vi "NiSwitch RouteTriggerInput.vi"(6 "contextId":T1, 8 "error in":errorcluster, 9 "timeout (ms)":i32=-1, 10 "Request Data":T3, 11 "gRPC ID":T1) -> (0 "error out":errorcluster, 2 "Response Data":T2, 3 "gRPC ID out":T1)   [LabVIEW 2021, in "NI Switch_client.lvlib"]
uses:
  NI Switch_client.lvlib
  <vilib>/gRPC/LabVIEW gRPC Library/Shared/grpcId.ctl
  RPC Messages/niswitch_grpc_RouteTriggerInputRequest.ctl
  RPC Messages/niswitch_grpc_RouteTriggerInputRequest_trigger_input_connector_enum/niswitch_grpc_RouteTriggerInputRequest_trigger_input_connector_enum.lvclass
  RPC Messages/niswitch_grpc_RouteTriggerInputRequest_trigger_input_bus_line_enum/niswitch_grpc_RouteTriggerInputRequest_trigger_input_bus_line_enum.lvclass
  RPC Messages/nidevice_grpc_Session.ctl
  RPC Messages/niswitch_grpc_RouteTriggerInputResponse.ctl
  RPC Messages/niswitch_grpc_RouteTriggerInputResponse_Flat.ctl
  RPC Messages/niswitch_grpc_RouteTriggerInputRequest_trigger_input_connector_enum/niswitch_grpc_RouteTriggerInputRequest_trigger_input_connector_enum.lvclass/niswitch_grpc_RouteTriggerInputRequest_trigger_input_connector_enum.ctl
  RPC Messages/niswitch_grpc_RouteTriggerInputRequest_trigger_input_bus_line_enum/niswitch_grpc_RouteTriggerInputRequest_trigger_input_bus_line_enum.lvclass/niswitch_grpc_RouteTriggerInputRequest_trigger_input_bus_line_enum.ctl
  14035477-4c25-4107-8ed5-d0c4ef420ce5.vi
  RPC Messages/RichToFlatnidevice_grpc_Session.vi
  RPC Messages/niswitch_grpc_RouteTriggerInputRequest_trigger_input_connector_enum/GetActiveFieldIndex.vi
  RPC Messages/niswitch_grpc_RouteTriggerInputRequest_trigger_input_connector_enum/Gettrigger_input_connector.vi
  RPC Messages/niswitch_grpc_RouteTriggerInputRequest_trigger_input_connector_enum/Gettrigger_input_connector_raw.vi
  RPC Messages/niswitch_grpc_RouteTriggerInputRequest_trigger_input_bus_line_enum/GetActiveFieldIndex.vi
  RPC Messages/niswitch_grpc_RouteTriggerInputRequest_trigger_input_bus_line_enum/Gettrigger_input_bus_line.vi
  RPC Messages/niswitch_grpc_RouteTriggerInputRequest_trigger_input_bus_line_enum/Gettrigger_input_bus_line_raw.vi
  <vilib>/gRPC/LabVIEW gRPC Library/Shared/TranslateGrpcError.vi
  <vilib>/gRPC/LabVIEW gRPC Library/Shared/Wait On Occurrence Wrapper.vi
  <vilib>/gRPC/LabVIEW gRPC Library/Shared/Wait On Occurence.vi
  <vilib>/gRPC/LabVIEW gRPC Library/Server API/Server/Get Server DLL Path.vi
  <vilib>/Utility/error.llb/Error Cluster From Error Code.vi
  <vilib>/Utility/config.llb/Open Config Data.vi
  <vilib>/Utility/config.llb/Write Key.vi
  <vilib>/Utility/config.llb/Write Key (Boolean).vi
  <vilib>/Utility/config.llb/Not A Config Data Refnum.vi
  <vilib>/Utility/config.llb/Read Key.vi
  <vilib>/Utility/config.llb/Read Key (Boolean).vi
  <vilib>/Utility/config.llb/Close Config Data.vi
  <vilib>/gRPC/LabVIEW gRPC Library/grpc-lvsupport-release.lvlib
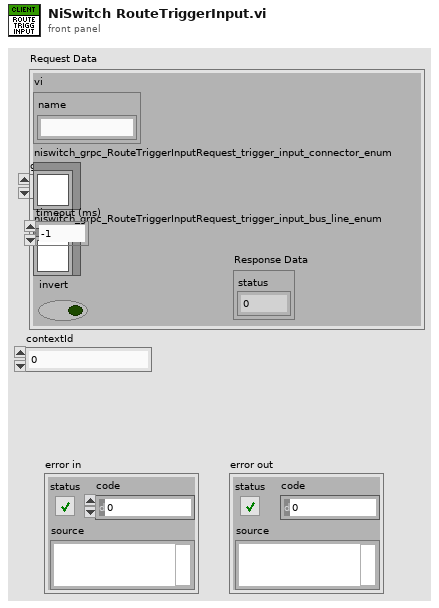
[diagram p1: front panel]
types:
  T1 = typedef "grpc-lvsupport-release.lvlib/grpcId.ctl" = u64
  T2 = typedef "NI Switch_client.lvlib/niswitch_grpc_RouteTriggerInputResponse.ctl" = cluster{"status":i32}
  T3 = typedef "NI Switch_client.lvlib/niswitch_grpc_RouteTriggerInputRequest.ctl" = cluster{"vi":T4, "niswitch_grpc_RouteTriggerInputRequest_trigger_input_connector_enum":refnum<class "niswitch_grpc_RouteTriggerInputRequest_trigger_input_connector_enum.lvclass">, "niswitch_grpc_RouteTriggerInputRequest_trigger_input_bus_line_enum":refnum<class "niswitch_grpc_RouteTriggerInputRequest_trigger_input_bus_line_enum.lvclass">, "invert":bool}
  T4 = typedef "NI Switch_client.lvlib/nidevice_grpc_Session.ctl" = cluster{"name":string}
  T5 = typedef "NI Switch_client.lvlib/niswitch_grpc_RouteTriggerInputResponse_Flat.ctl" = cluster{"status":i32}
  T6 = typedef "NI Switch_client.lvlib/niswitch_grpc_RouteTriggerInputRequest_Flat.ctl" = cluster{"vi":T7, "niswitch_grpc_RouteTriggerInputRequest_trigger_input_connector_enum_selected_index":i32, "trigger_input_connector":T8, "trigger_input_connector_raw":i32, "niswitch_grpc_RouteTriggerInputRequest_trigger_input_bus_line_enum_selected_index":i32, "trigger_input_bus_line":T8, "trigger_input_bus_line_raw":i32, "invert":bool}
  T7 = typedef "NI Switch_client.lvlib/nidevice_grpc_Session_Flat.ctl" = cluster{"name":string}
  T8 = typedef "NI Switch_client.lvlib/niswitch_grpc_TriggerInput.ctl" = enum32{"TRIGGER_INPUT_UNSPECIFIED", "TRIGGER_INPUT_NISWITCH_VAL_IMMEDIATE", "TRIGGER_INPUT_NISWITCH_VAL_EXTERNAL", "TRIGGER_INPUT_NISWITCH_VAL_SOFTWARE_TRIG", "TRIGGER_INPUT_NISWITCH_VAL_TTL0", "TRIGGER_INPUT_NISWITCH_VAL_TTL1", "TRIGGER_INPUT_NISWITCH_VAL_TTL2", "TRIGGER_INPUT_NISWITCH_VAL_TTL3", "TRIGGER_INPUT_NISWITCH_VAL_TTL4", "TRIGGER_INPUT_NISWITCH_VAL_TTL5", "TRIGGER_INPUT_NISWITCH_VAL_TTL6", "TRIGGER_INPUT_NISWITCH_VAL_TTL7", "TRIGGER_INPUT_NISWITCH_VAL_PXI_STAR", "TRIGGER_INPUT_NISWITCH_VAL_REARCONNECTOR", "TRIGGER_INPUT_NISWITCH_VAL_FRONTCONNECTOR", "TRIGGER_INPUT_NISWITCH_VAL_REARCONNECTOR_MODULE1", "TRIGGER_INPUT_NISWITCH_VAL_REARCONNECTOR_MODULE2", "TRIGGER_INPUT_NISWITCH_VAL_REARCONNECTOR_MODULE3", "TRIGGER_INPUT_NISWITCH_VAL_REARCONNECTOR_MODULE4", "TRIGGER_INPUT_NISWITCH_VAL_REARCONNECTOR_MODULE5", "TRIGGER_INPUT_NISWITCH_VAL_REARCONNECTOR_MODULE6", "TRIGGER_INPUT_NISWITCH_VAL_REARCONNECTOR_MODULE7", "TRIGGER_INPUT_NISWITCH_VAL_REARCONNECTOR_MODULE8", "TRIGGER_INPUT_NISWITCH_VAL_REARCONNECTOR_MODULE9", "TRIGGER_INPUT_NISWITCH_VAL_REARCONNECTOR_MODULE10", "TRIGGER_INPUT_NISWITCH_VAL_REARCONNECTOR_MODULE11", "TRIGGER_INPUT_NISWITCH_VAL_REARCONNECTOR_MODULE12", "TRIGGER_INPUT_NISWITCH_VAL_FRONTCONNECTOR_MODULE1", "TRIGGER_INPUT_NISWITCH_VAL_FRONTCONNECTOR_MODULE2", "TRIGGER_INPUT_NISWITCH_VAL_FRONTCONNECTOR_MODULE3", "TRIGGER_INPUT_NISWITCH_VAL_FRONTCONNECTOR_MODULE4", "TRIGGER_INPUT_NISWITCH_VAL_FRONTCONNECTOR_MODULE5", "TRIGGER_INPUT_NISWITCH_VAL_FRONTCONNECTOR_MODULE6", "TRIGGER_INPUT_NISWITCH_VAL_FRONTCONNECTOR_MODULE7", "TRIGGER_INPUT_NISWITCH_VAL_FRONTCONNECTOR_MODULE8", "TRIGGER_INPUT_NISWITCH_VAL_FRONTCONNECTOR_MODULE9", "TRIGGER_INPUT_NISWITCH_VAL_FRONTCONNECTOR_MODULE10", "TRIGGER_INPUT_NISWITCH_VAL_FRONTCONNECTOR_MODULE11", "TRIGGER_INPUT_NISWITCH_VAL_FRONTCONNECTOR_MODULE12"}
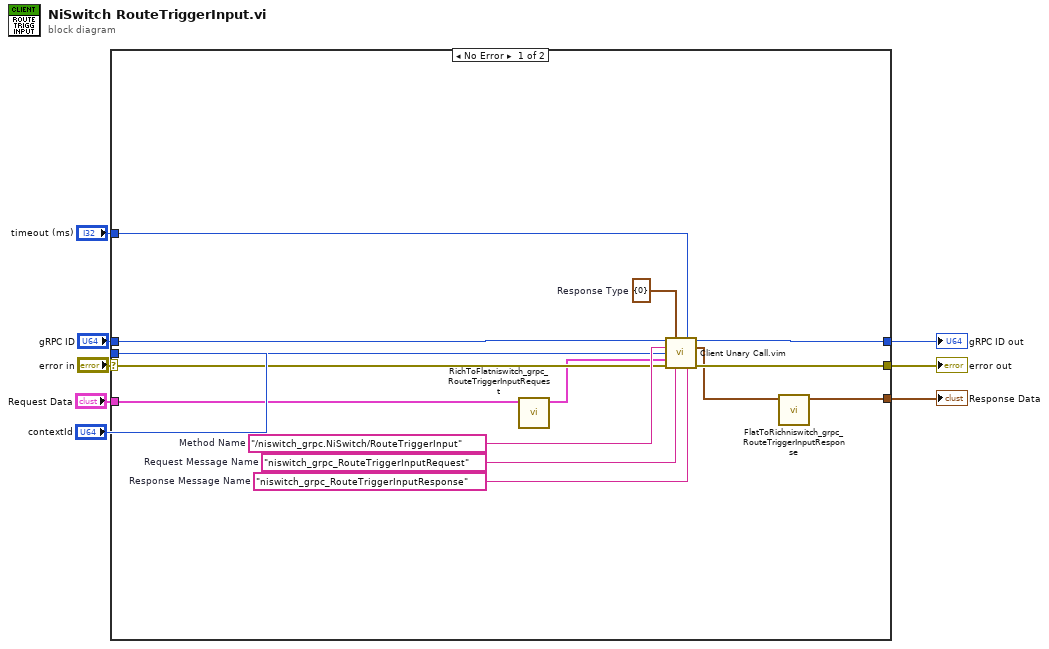
[diagram p0: block diagram]
diagram:
  n1 = case shown="No Error" "error in" {
    selector: "error in" -> [w18 w23]
    tunnel: [w17 w23] -> w7
    tunnel: "gRPC ID" -> [w16 w24]
    tunnel: [w15 w24] -> w5
    tunnel: "Request Data" -> [w12 _]
    tunnel: [w9 _] -> w3
    tunnel: "timeout (ms)" -> [w14 _]
    tunnel: "contextId" -> [w13 _]
    frame No Error {
      w19 = "niswitch_grpc_RouteTriggerInputResponse"  # Response Message Name
      w20 = "niswitch_grpc_RouteTriggerInputRequest"  # Request Message Name
      w21 = T5 {"status"=0}  # Response Type
      w22 = "/niswitch_grpc.NiSwitch/RouteTriggerInput"  # Method Name
      n2 = call "RichToFlatniswitch_grpc_RouteTriggerInputRequest.vi"("InputCluster"=w12) -> ("OutputCluster"=w11:T6)  [unwired: 10 in]
      n3 = call "Client Unary Call.vim"("ClientID in"=w16, "Response Type"=w21, "timeout (ms)"=w14, "Method Name"=w22, "contextId"=w13, "Request Data"=w11, "error in"=w18, "Request Message Name"=w20, "Response Message Name"=w19) -> ("ClientID out"=w15:u64, "Response Data"=w10:T5, "error out"=w17:errorcluster)  [unwired: 4 in]
      n4 = call "FlatToRichniswitch_grpc_RouteTriggerInputResponse.vi"("InputCluster"=w10) -> ("OutputCluster"=w9:T2)  [unwired: 10 in]
    }
    frame Error {
    }
  }
  "error out" <- w7
  "gRPC ID out" <- w5
  "Response Data" <- w3
